vi "Set Windows Position.vi"(7 "Position":T1(ring), 8 "error in (no error)":errorcluster, 9 "uFlags":string(combo), 10 "hWndInsertAfter":string(combo), 11 "hWnd":u32) -> (0 "error out":errorcluster, 3 "hWnd out":u32)   [LabVIEW 2019, in "Test Bench Tools.lvlib"]
uses:
  Test Bench Tools.lvlib
  user32.dll
panel:
  out "ok?":bool
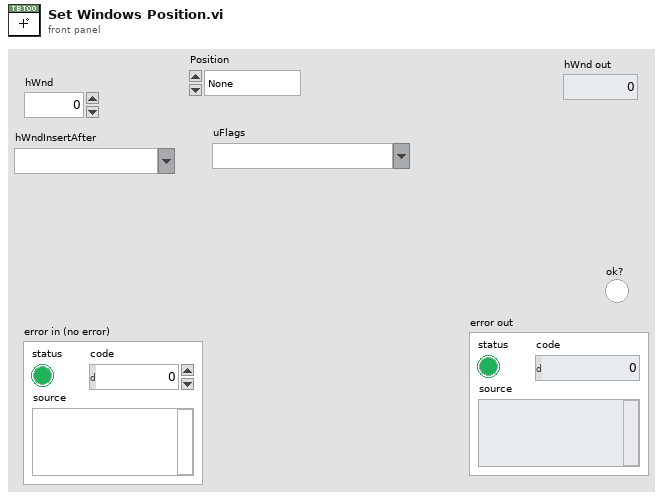
[diagram p1: front panel]
types:
  T1 = enum16{"None", "Top", "Bottom", "Left", "Right", "Left-Top", "Left-Bottom", "Right-Top", "Right-Bottom"}
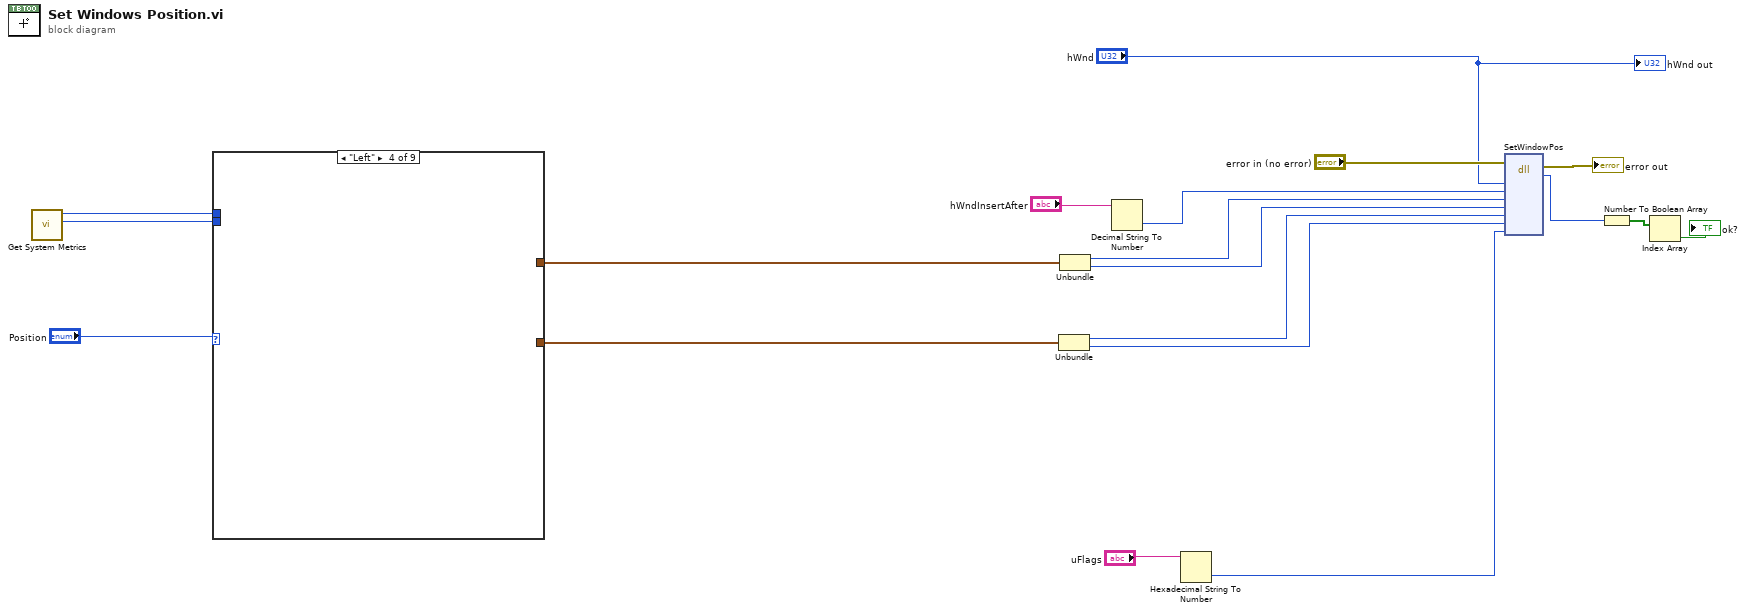
[diagram p0: block diagram]
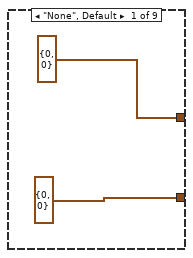
[diagram p2: hidden frame]
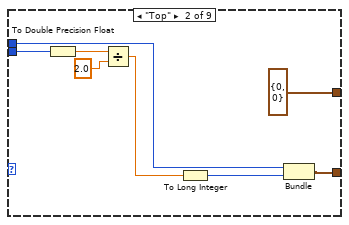
[diagram p3: hidden frame]
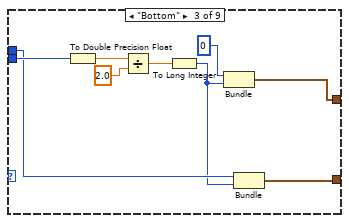
[diagram p4: hidden frame]
diagram:
  n1 = call "Get System Metrics.vi"() -> ("Y"=w1:i32, "X"=w2:i32)  [unwired: 9 in, 1 out]
  n2 = case shown="\"Left\"" "Position" {
    tunnel: [cluster{"cx":i32, "cy":i32} {"cx"=0, "cy"=0} ("Size") w23 w32 _ _ _ _ _ _] -> w4
    tunnel: [cluster{"X":i32, "Y":i32} {"X"=0, "Y"=0} ("Position") cluster{"X":i32, "Y":i32} {"X"=0, "Y"=0} ("Position") w34 _ _ _ _ _ _] -> w3
    tunnel: w2 -> [_ w28 w33 _ _ _ _ _ _]
    tunnel: w1 -> [_ w27 w36 _ _ _ _ _ _]
    frame "None", Default {
    }
    frame "Top" {
      n3 = To Double Precision Float(number=w27) -> (double precision float=w22:dbl)
      n4 = Divide(x=w22, y=2.0) -> (x/y=w25:dbl)
      n5 = To Long Integer(number=w25) -> (32bit integer=w24:i32)
      n6 = Bundle("X"=w28, w24) -> (w23:cluster{"X":i32, i32})  [unwired: 1 in]
    }
    frame "Bottom" {
      n7 = To Double Precision Float(number=w36) -> (double precision float=w37:dbl)
      n8 = Divide(x=w37, y=2.0) -> (x/y=w35:dbl)
      n9 = To Long Integer(number=w35) -> (32bit integer=w30:i32)
      n10 = Bundle("X"=0, w30) -> (w34:cluster{"X":i32, i32})  [unwired: 1 in]
      n11 = Bundle("X"=w33, w30) -> (w32:cluster{"X":i32, i32})  [unwired: 1 in]
    }
    frame "Left" {
    }
    frame "Right" {
    }
    frame "Left-Top" {
    }
    frame "Left-Bottom" {
    }
    frame "Right-Top" {
    }
    frame "Right-Bottom" {
    }
  }
  n12 = Unbundle(w4) -> ("X"=w15:i32, "cy"=w14:i32)
  n13 = Unbundle(w3) -> ("X"=w17:i32, "Y"=w16:i32)
  n14 = Decimal String To Number(string="hWndInsertAfter") -> (number=w12:i32)  [unwired: 2 in, 1 out]
  n15 = Hexadecimal String To Number(string="uFlags") -> (number=w10:u32)  [unwired: 2 in, 1 out]
  n16 = dll-call lib="USER32.DLL" fn="SetWindowPos"(error in="error in (no error)", "hWnd"="hWnd", "hWndInsertAfter"=w12, "left"=w17, "top"=w16, "width"=w15, "height"=w14, "fuFlags"=w10) -> (error out=→"error out":errorcluster, "error"=w8:i32)  [unwired: 9 in, 1 out]
  n17 = Number To Boolean Array(number=w8) -> (Boolean array=w7:bool[])
  n18 = Index Array(array=w7) -> (element=→"ok?":bool)  [unwired: 1 in]
  "hWnd out" <- "hWnd"
